vi "Config - Search.vi"(8 "error in (no error)":errorcluster, 10 "Account Number":u32, 11 "Data Records":T1[](array[typedef])) -> (0 "error out":errorcluster, 1 "Found?":bool, 2 "Data Record":T1)   [LabVIEW 2017]
doc: "Search data record from Array by Account number."
uses:
  Controls/Config Data Record.ctl
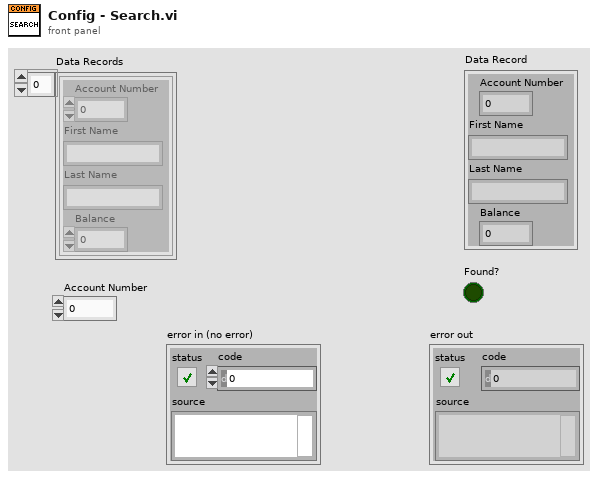
[diagram p1: front panel]
types:
  T1 = typedef "Config Data Record.ctl" = cluster{"Account Number":u32, "First Name":string, "Last Name":string, "Balance":dbl}
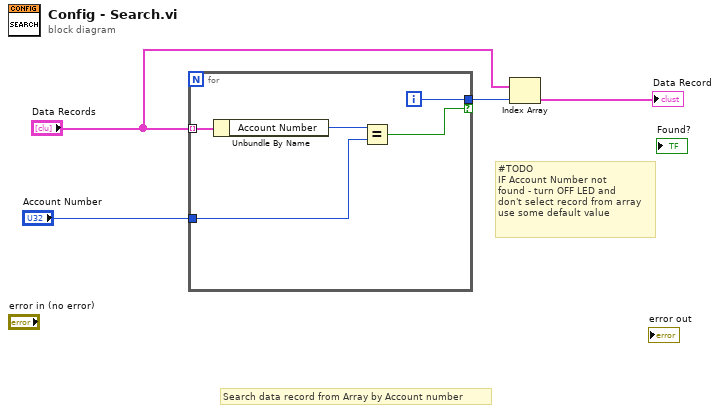
[diagram p0: block diagram]
diagram:
  # "#TODO\nIF Account Number not\nfound - turn OFF LED and\ndon't select record from array\nuse some default value"
  # "Search data record from Array by Account number"
  n1 = for {
    tunnel: "Data Records" -> [w9] mode=indexing
    tunnel: "Account Number" -> [w7]
    tunnel: [w6] -> w2 if=w5
    i -> [w6]
    n2 = Unbundle By Name(w9) -> ("Account Number"=w8:u32)
    n3 = Equal?(x=w8, y=w7) -> (x = y?=w5:bool)
  }
  n4 = Index Array(array="Data Records", index=w2) -> (element=→"Data Record":T1)
